vi "PLC to MES monitor.vi"(0 "UTP IO Session in":T1, 5 "Sequence Context In":refnum<k7>, 7 "Logged In":bool, 9 "Packaging Performed":bool, 11 "error in":errorcluster) -> (4 "UTP IO Session out":T1, 15 "error out":errorcluster)   [LabVIEW 2023]
uses:
  <vilib>/Noffz/UTP IO/UTP IO Library/Typedefs/Session Handle.ctl
  <vilib>/Noffz/UTP IO/UTP IO Library/UTP IO Pool Session.lvclass
  MES/RequestData.ctl
  5ea416fa-7da9-46cf-b64f-edb3a1b9c4c5.vi
  <vilib>/Noffz/UTP IO/UTP IO Library/methods/poly/plc/Read PLC Variable (Boolean).vi
  <vilib>/Noffz/UTP IO/UTP IO Library/methods/poly/plc/Write PLC Variable (Boolean).vi
  <vilib>/Noffz/UTP IO/UTP IO Library/methods/poly/plc/Write PLC Variable (I16).vi
  <vilib>/addons/TestStand/_TSUtility.llb/TestStand - Get Property Value (Boolean).vi
  <vilib>/addons/TestStand/_TSUtility.llb/TestStand - Get Property Value (String).vi
panel:
  in  "stop":bool
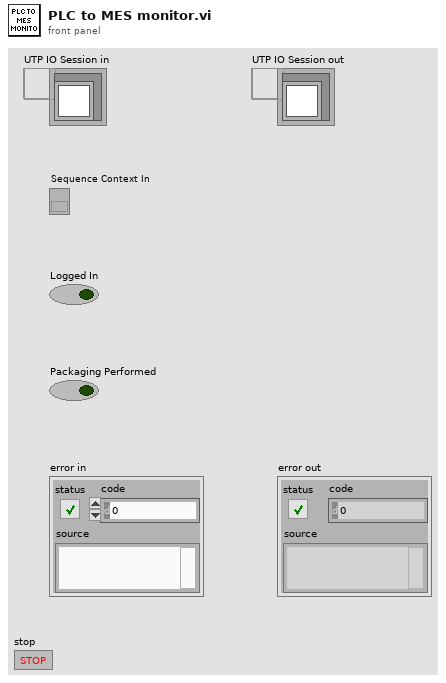
[diagram p1: front panel]
types:
  T1 = typedef "UTP IO Library.lvlib/UTP IO Pool Session.lvclass/Session Handle.ctl" = refnum<data-value>
  T2 = typedef "RequestData.ctl" = cluster{"SOAP":cluster{"HuNo":string, "MaterialCode":string, "Mode":i32, "Operator":string, "PackingInstructions":string, "ProductionVersion":string, "SerialNo":string}, "HU Validation":cluster{"MaterialCode":string, "Operator":string, "SerialNo":string}, "Login":cluster{"EquipmentCode":string, "Mode":i32, "Operator":string}}
  T3 = typedef "TestStand - Status Monitor.ctl" = cluster{"Sequence Context":refnum<k7>, "Execution":refnum<k7>, "Termination Monitor":refnum<k7>}
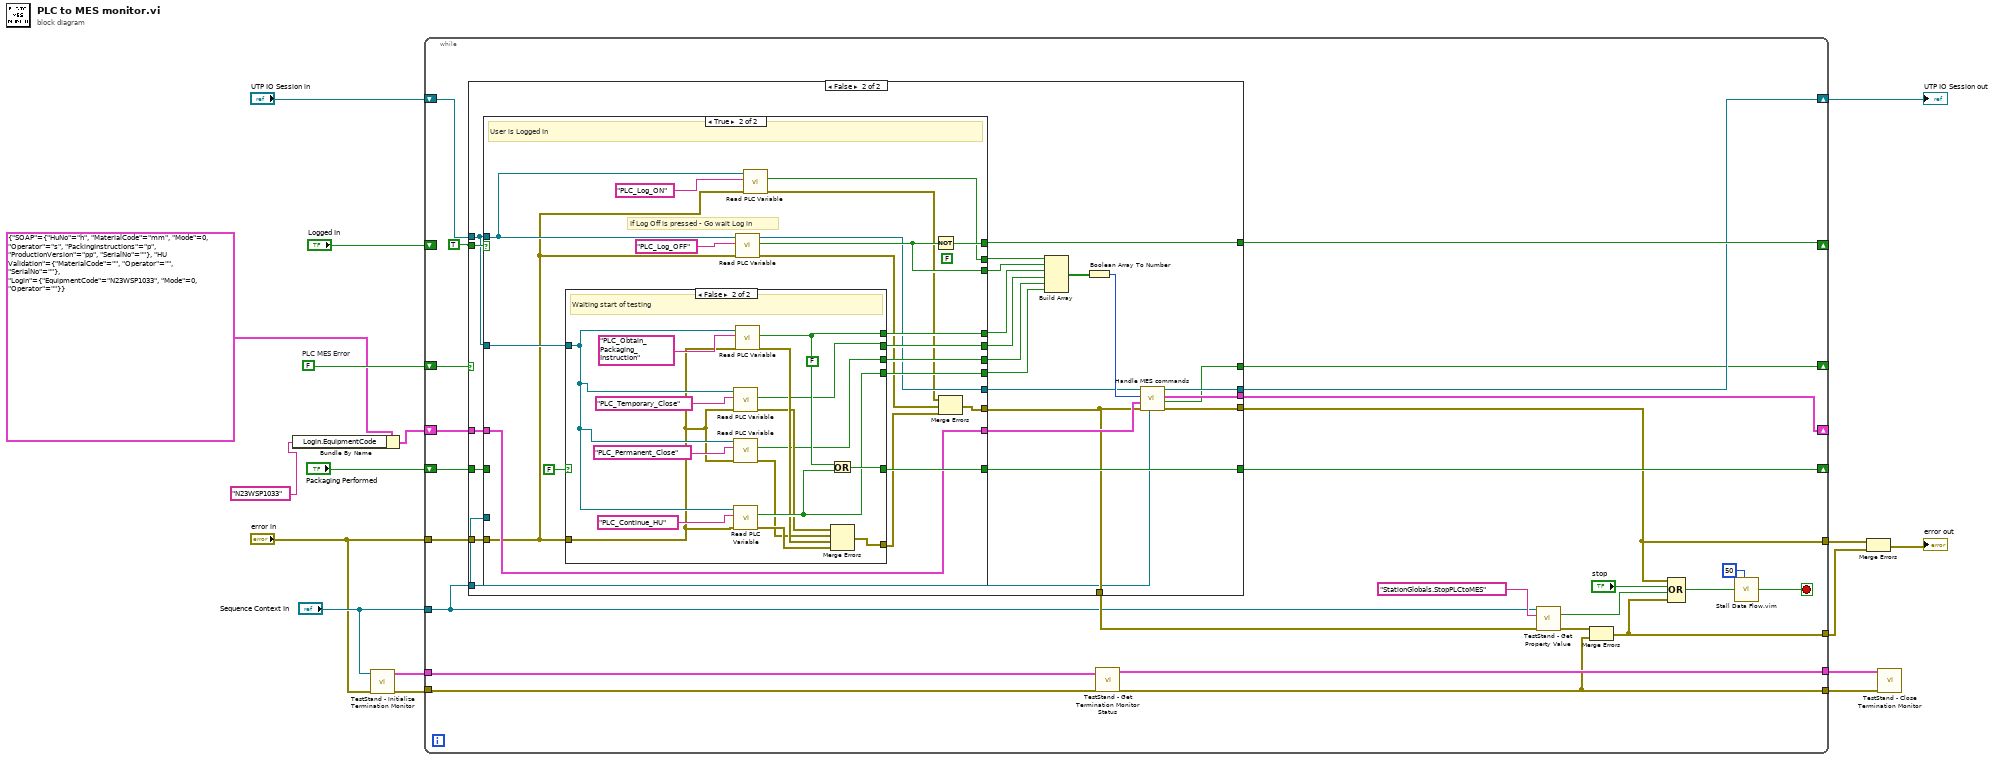
[diagram p0: block diagram]
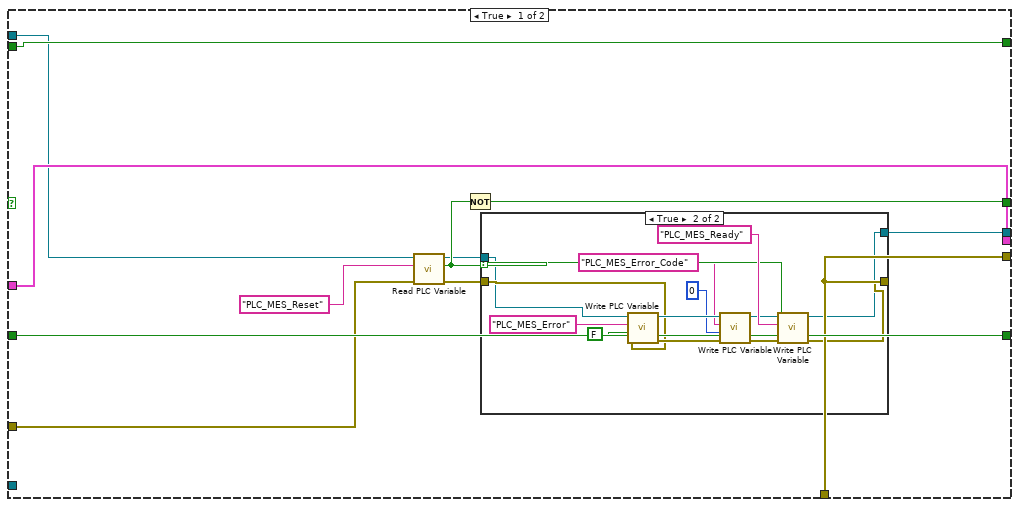
[diagram p2: hidden frame]
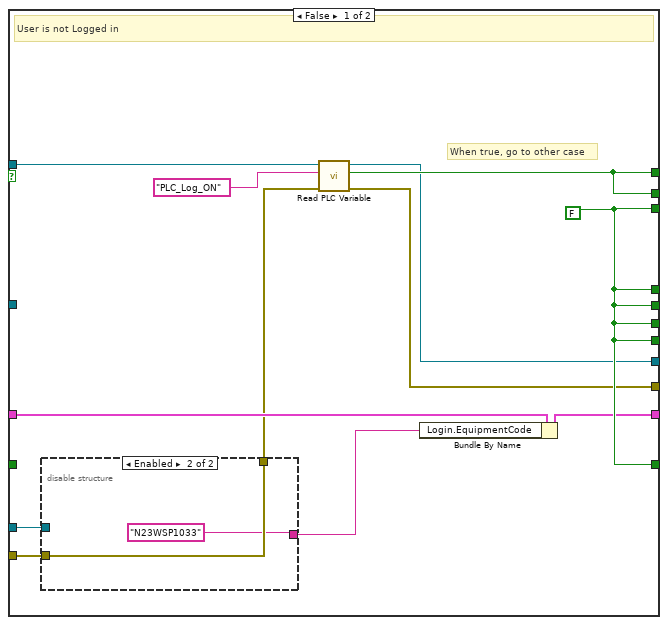
[diagram p4: hidden frame]
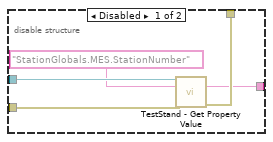
[diagram p5: hidden frame]
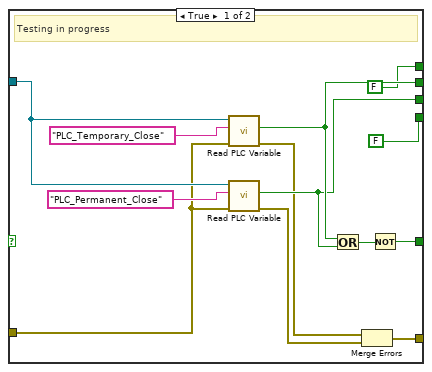
[diagram p6: hidden frame]
diagram:
  w4 = FALSE  # PLC MES Error
  n1 = Bundle By Name(cluster=T2 {"SOAP"={"HuNo"="h", "MaterialCode"="mm", "Mode"=0, "Operator"="s", "PackingInstructions"="p", "ProductionVersion"="pp", "SerialNo"=""}, "HU Validation"={"MaterialCode"="", "Operator"="", "SerialNo"=""}, "Login"={"EquipmentCode"="N23WSP1033", "Mode"=0, "Operator"=""}} ("RequestData"), "Login.EquipmentCode"="N23WSP1033" ("Value")) -> (w2:T2)
  n2 = call <vilib>:"TestStand - Initialize Termination Monitor.vi"("error in (no error)"="error in", "Sequence Context In"="Sequence Context In") -> ("error out"=w13:errorcluster, "Status Monitor Out"=w11:T3)  [unwired: 8 in]
  n3 = while {
    shift-right: [w28] -> w16
    shift-left: "UTP IO Session in" -> [w29]
    shift-right: [w43] -> _
    shift-left: "Logged In" -> [_]
    shift-right: [w41] -> _
    shift-left: "Packaging Performed" -> [w42]
    tunnel: w13 -> [w40]
    tunnel: [w32] -> w12
    tunnel: w11 -> [w39]
    tunnel: [w38] -> w10
    tunnel: "Sequence Context In" -> [w21]
    tunnel: "error in" -> [w31]
    tunnel: [w23] -> w7
    tunnel: [w30] -> w5
    shift-right: [w26] -> _
    shift-left: w2 -> [w27]
    shift-right: [w19] -> _
    shift-left: w4 -> [w20]
    stop <- w25 stop-if-true
    n4 = case shown="False" w20 {
      tunnel: TRUE ("Logged In") -> [w55 w94]
      tunnel: [w55 w93] -> w43
      tunnel: w42 -> [w53 w89]
      tunnel: [w53 w88] -> w41
      tunnel: w31 -> [w51 w82]
      tunnel: w29 -> [w52 w81]
      tunnel: [w46 w79] -> w28
      tunnel: w27 -> [w54 w77]
      tunnel: [w54 w76] -> w26
      tunnel: [w44 w75] -> w23
      tunnel: [w44 w74] -> w22
      tunnel: w21 -> [_ w73]
      tunnel: [w49 w72] -> w19
      frame True {
        n5 = call-poly <vilib>:"Read PLC Variable.vi"("error in (no error)"=w51, "variable name"="PLC_MES_Reset", "UTP IO Session in"=w52) -> ("error out"=w45:errorcluster, "value"=w48:bool, "UTP IO Session out"=w47:T1)  [unwired: 6 in]
        n6 = Not(x=w48) -> (.not. x?=w49:bool)
        n7 = case shown="True" w48 {
          selector: w48 -> [_ w70]
          tunnel: w47 -> [w57 w62]
          tunnel: [w57 w61] -> w46
          tunnel: w45 -> [w56 w65]
          tunnel: [w56 w63] -> w44
          frame False {
          }
          frame True {
            n8 = call-poly <vilib>:"Write PLC Variable.vi"("error in (no error)"=w65, "value"=FALSE, "variable name"="PLC_MES_Error", "UTP IO Session in"=w62) -> ("error out"=w68:errorcluster, "UTP IO Session out"=w69:T1)  [unwired: 6 in]
            n9 = call-poly <vilib>:"Write PLC Variable.vi"("error in (no error)"=w68, "value"=i16 0, "variable name"="PLC_MES_Error_Code", "UTP IO Session in"=w69) -> ("error out"=w64:errorcluster, "UTP IO Session out"=w58:T1)  [unwired: 6 in]
            n10 = call-poly <vilib>:"Write PLC Variable.vi"("error in (no error)"=w64, "value"=w70, "variable name"="PLC_MES_Ready", "UTP IO Session in"=w58) -> ("error out"=w63:errorcluster, "UTP IO Session out"=w61:T1)  [unwired: 6 in]
          }
        }
      }
      frame False {
        n11 = case shown="True" w94 {
          tunnel: w81 -> [w105 w118]
          tunnel: [w104 w132] -> w93
          tunnel: w81 -> [_ w131]
          tunnel: [w103 w130] -> w90
          tunnel: [w104 w115] -> w91
          tunnel: w89 -> [_ _]
          tunnel: [w103 w129] -> w87
          tunnel: [w103 w128] -> w86
          tunnel: [w103 w127] -> w85
          tunnel: [w103 w126] -> w88
          tunnel: [w103 w125] -> w84
          tunnel: w82 -> [w98 w117]
          tunnel: [w102 w124] -> w74
          tunnel: [w101 w121] -> w80
          tunnel: [w96 w120] -> w78
          tunnel: w77 -> [w100 w120]
          tunnel: w73 -> [w99 _]
          frame False {
            w103 = FALSE ("value")
            # "When true, go to other case"
            # "User is not Logged in"
            n12 = disable-structure shown="Enabled" {
              disable-tunnel: w99 -> [w111 _]
              disable-tunnel: w98 -> [w110 w113]
              disable-tunnel: [w108 w113] -> w97
              disable-tunnel: [w107 "N23WSP1033" ("Value")] -> w95
              frame Disabled {
                n13 = call-poly <vilib>:"TestStand - Get Property Value.vi"("Sequence Context In"=w111, "Lookup String"="StationGlobals.MES.StationNumber", "error in (no error)"=w110) -> ("Value"=w107:string, "error out"=w108:errorcluster)  [unwired: 10 in, 1 out]
              }
              frame Enabled {
              }
            }
            n14 = call-poly <vilib>:"Read PLC Variable.vi"("error in (no error)"=w97, "variable name"="PLC_Log_ON", "UTP IO Session in"=w105) -> ("error out"=w102:errorcluster, "value"=w104:bool, "UTP IO Session out"=w101:T1)  [unwired: 6 in]
            n15 = Bundle By Name(cluster=w100, "Login.EquipmentCode"=w95) -> (w96:T2)
          }
          frame True {
            (unwired) FALSE ("value")
            # "If Log Off is pressed - Go wait Log in"
            # "User is Logged In"
            n16 = case shown="False" FALSE {
              tunnel: w131 -> [w144 w152]
              tunnel: [FALSE ("value") w159] -> w129
              tunnel: [w143 w148] -> w128
              tunnel: [w142 w147] -> w127
              tunnel: [w140 w160] -> w126
              tunnel: [FALSE ("value") w158] -> w125
              tunnel: w117 -> [w137 w151]
              tunnel: [w134 w157] -> w123
              frame True {
                # "Testing in progress"
                n17 = call-poly <vilib>:"Read PLC Variable.vi"("error in (no error)"=w137, "variable name"="PLC_Temporary_Close", "UTP IO Session in"=w144) -> ("error out"=w136:errorcluster, "value"=w143:bool)  [unwired: 6 in, 1 out]
                n18 = call-poly <vilib>:"Read PLC Variable.vi"("error in (no error)"=w137, "variable name"="PLC_Permanent_Close", "UTP IO Session in"=w144) -> ("error out"=w135:errorcluster, "value"=w142:bool)  [unwired: 6 in, 1 out]
                n19 = Or(x=w143, y=w142) -> (x .or. y?=w141:bool)
                n20 = Merge Errors(w136, w135) -> (w134:errorcluster)
                n21 = Not(x=w141) -> (.not. x?=w140:bool)
              }
              frame False {
                (unwired) FALSE ("value")
                # "Waiting start of testing"
                n22 = call-poly <vilib>:"Read PLC Variable.vi"("error in (no error)"=w151, "variable name"="PLC_Temporary_Close", "UTP IO Session in"=w152) -> ("error out"=w150:errorcluster, "value"=w148:bool)  [unwired: 6 in, 1 out]
                n23 = call-poly <vilib>:"Read PLC Variable.vi"("error in (no error)"=w151, "variable name"="PLC_Permanent_Close", "UTP IO Session in"=w152) -> ("error out"=w149:errorcluster, "value"=w147:bool)  [unwired: 6 in, 1 out]
                n24 = call-poly <vilib>:"Read PLC Variable.vi"("error in (no error)"=w151, "variable name"="PLC_Continue_HU", "UTP IO Session in"=w152) -> ("error out"=w155:errorcluster, "value"=w158:bool)  [unwired: 6 in, 1 out]
                n25 = call-poly <vilib>:"Read PLC Variable.vi"("error in (no error)"=w151, "variable name"="PLC_Obtain_Packaging_Instruction", "UTP IO Session in"=w152) -> ("error out"=w156:errorcluster, "value"=w159:bool)  [unwired: 6 in, 1 out]
                n26 = Or(x=w159, y=w158) -> (x .or. y?=w160:bool)
                n27 = Merge Errors(w150, w149, w156, w155) -> (w157:errorcluster)
              }
            }
            n28 = call-poly <vilib>:"Read PLC Variable.vi"("error in (no error)"=w117, "variable name"="PLC_Log_OFF", "UTP IO Session in"=w118) -> ("error out"=w122:errorcluster, "value"=w130:bool, "UTP IO Session out"=w121:T1)  [unwired: 6 in]
            n29 = call-poly <vilib>:"Read PLC Variable.vi"("error in (no error)"=w117, "variable name"="PLC_Log_ON", "UTP IO Session in"=w118) -> ("error out"=w116:errorcluster, "value"=w115:bool)  [unwired: 6 in, 1 out]
            n30 = Not(x=w130) -> (.not. x?=w132:bool)
            n31 = Merge Errors(w116, w122, w123) -> (w124:errorcluster)
          }
        }
        n32 = Build Array(w91, w90, w87, w86, w85, w84) -> (w92:bool[])
        n33 = Boolean Array To Number(Boolean array=w92) -> (number=w83:u32)
        n34 = call "Handle MES commands.vi"("Sequence Context In"=w73, "error in (no error)"=w74, "RequestData in"=w78, "Request"=w83, "Data Value Reference in"=w80) -> ("error out"=w75:errorcluster, "PLC MES Error"=w72:bool, "RequestData out"=w76:T2, "Data Value Reference out"=w79:T1)  [unwired: 3 in]
      }
    }
    n35 = call <vilib>:"TestStand - Get Termination Monitor Status.vi"("error in (no error)"=w40, "Status Monitor In"=w39) -> ("error out"=w32:errorcluster, "Status Monitor Out"=w38:T3)  [unwired: 7 in, 1 out]
    n36 = call-poly <vilib>:"TestStand - Get Property Value.vi"("Sequence Context In"=w21, "Lookup String"="StationGlobals.StopPLCtoMES", "error in (no error)"=w22) -> ("Value"=w34:bool, "error out"=w33:errorcluster)  [unwired: 10 in, 1 out]
    n37 = Merge Errors(w33, w32) -> (w30:errorcluster)
    n38 = Compound Arithmetic op=OR(w23, "stop", w34, w30) -> (w35:bool)
    n39 = call "Stall Data Flow.vim"("value in"=w35, "milliseconds to wait"=u32 50) -> ("value out"=w25:bool)  [unwired: 1 out]
  }
  "UTP IO Session out" <- w16
  n40 = Merge Errors(w7, w5) -> (→"error out":errorcluster)
  n41 = call <vilib>:"TestStand - Close Termination Monitor.vi"("error in (no error)"=w12, "Status Monitor In"=w10) -> ()  [unwired: 9 in, 1 out]
